vi "Dashboard Main.vi"() -> ()   [LabVIEW 2013]
uses:
  <vilib>/Rock Robotics/WPI/Camera/WPI_CameraSettings Read MJPG.ctl
  <vilib>/Rock Robotics/WPI/Camera/WPI_CameraImageSize.ctl
  <vilib>/event_ctls.llb/eventvkey.ctl
panel:
  in  "Mode":T1(ring)=enum."Auto Disabled"
  out "Encoder Speed":dbl(graph)
  in  "Rec Mode":enum32{"Stop", "Record", "Playback"}(radio)
  out "Battery":sgl
  out "High Gear":bool
  out "Speed":dbl(knob) scale=0.0..25.0
  out "Dashboard Connected":bool
  in  "Tab Control":T2(tab)
  in  "Autonmous To Run":string(combo)
  in  "Autonmous mode":string
  in  "Editable":bool
  in  "Reload Autonmous text file":bool
  in  "Save Auto file back to text file":bool
  out "Camera":T3(plugin-control)
  in  "Reload Constants":bool
  out "Variable Names":string[](array[string])
  out "Array of Numbers":dbl[](array[numeric])
  in  "Listbox":i32(listbox)
  in  "Reset Gyro":bool
  out "gyroAngle":dbl
  # "CHANGE IP!!!!!!!!!!!!!!!!!!!!!!"
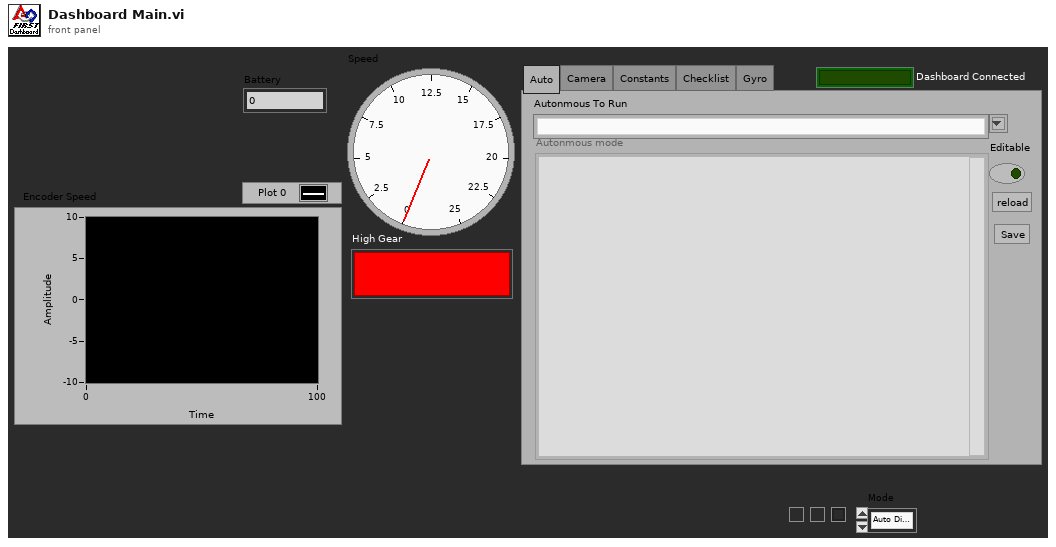
[diagram p1: front panel]
types:
  T1 = enum8{"Tele-Op Disabled", "Tele-Op Enabled", "Auto Disabled", "Auto Enabled", "Test Disabled", "Test Enabled", ""}
  T2 = enum32{"Auto", "Camera", "Constants", "Checklist", "Gyro"}
  T3 = typedef "IMAQ Image.ctl" = refnum<image>
  T4 = enum16{"None", "On Hover", "On Key Focus", "On Hover or Key Focus"}
  T5 = enum8{"Enabled", "Disabled", "Disabled and Grayed Out"}
  T6 = typedef "WPI_CameraSettings Read MJPG.ctl" = cluster{"fps":i32, "compression":i32, "Image Size":T7}
  T7 = typedef "WPI_CameraImageSize.ctl" = enum16{"640x480", "320x240", "160x120"}
  T8 = typedef "Image Type" = u32
  T9 = cluster{cluster{dbl, dbl}, cluster{dbl, dbl}, cluster{dbl, dbl}}
  T10 = cluster{"Digital Inputs":bool[], "Digital Outputs":bool[]}
  T11 = cluster{"Competition mode":bool, "Robot Link":bool, "Autonomous":bool, "Enabled":bool, "E-Stop":bool, "Simulated":bool, "TestMode":bool, "Docked Window":bool}
  T12 = typedef "eventvkey.ctl" = enum16{"ASCII", "Enter", "Return", "Shift", "Ctrl", "Alt", "Cmd", "Opt", "Caps", "NumLock", "Clear", "Break", "Up", "Down", "Left", "Right", "Insert", "Delete", "Home", "End", "PageUp", "PageDown", "Escape", "Help", "Pause", "ScrollLock", "F1", "F2", "F3", "F4", "F5", "F6", "F7", "F8", "F9", "F10", "F11", "F12", "F13", "F14", "F15", "F16", "F17", "F18", "F19", "F20", "F21", "F22", "F23", "F24", "Play", "VolumeUp", "VolumeDown", "Mute", "Two Byte Char"}
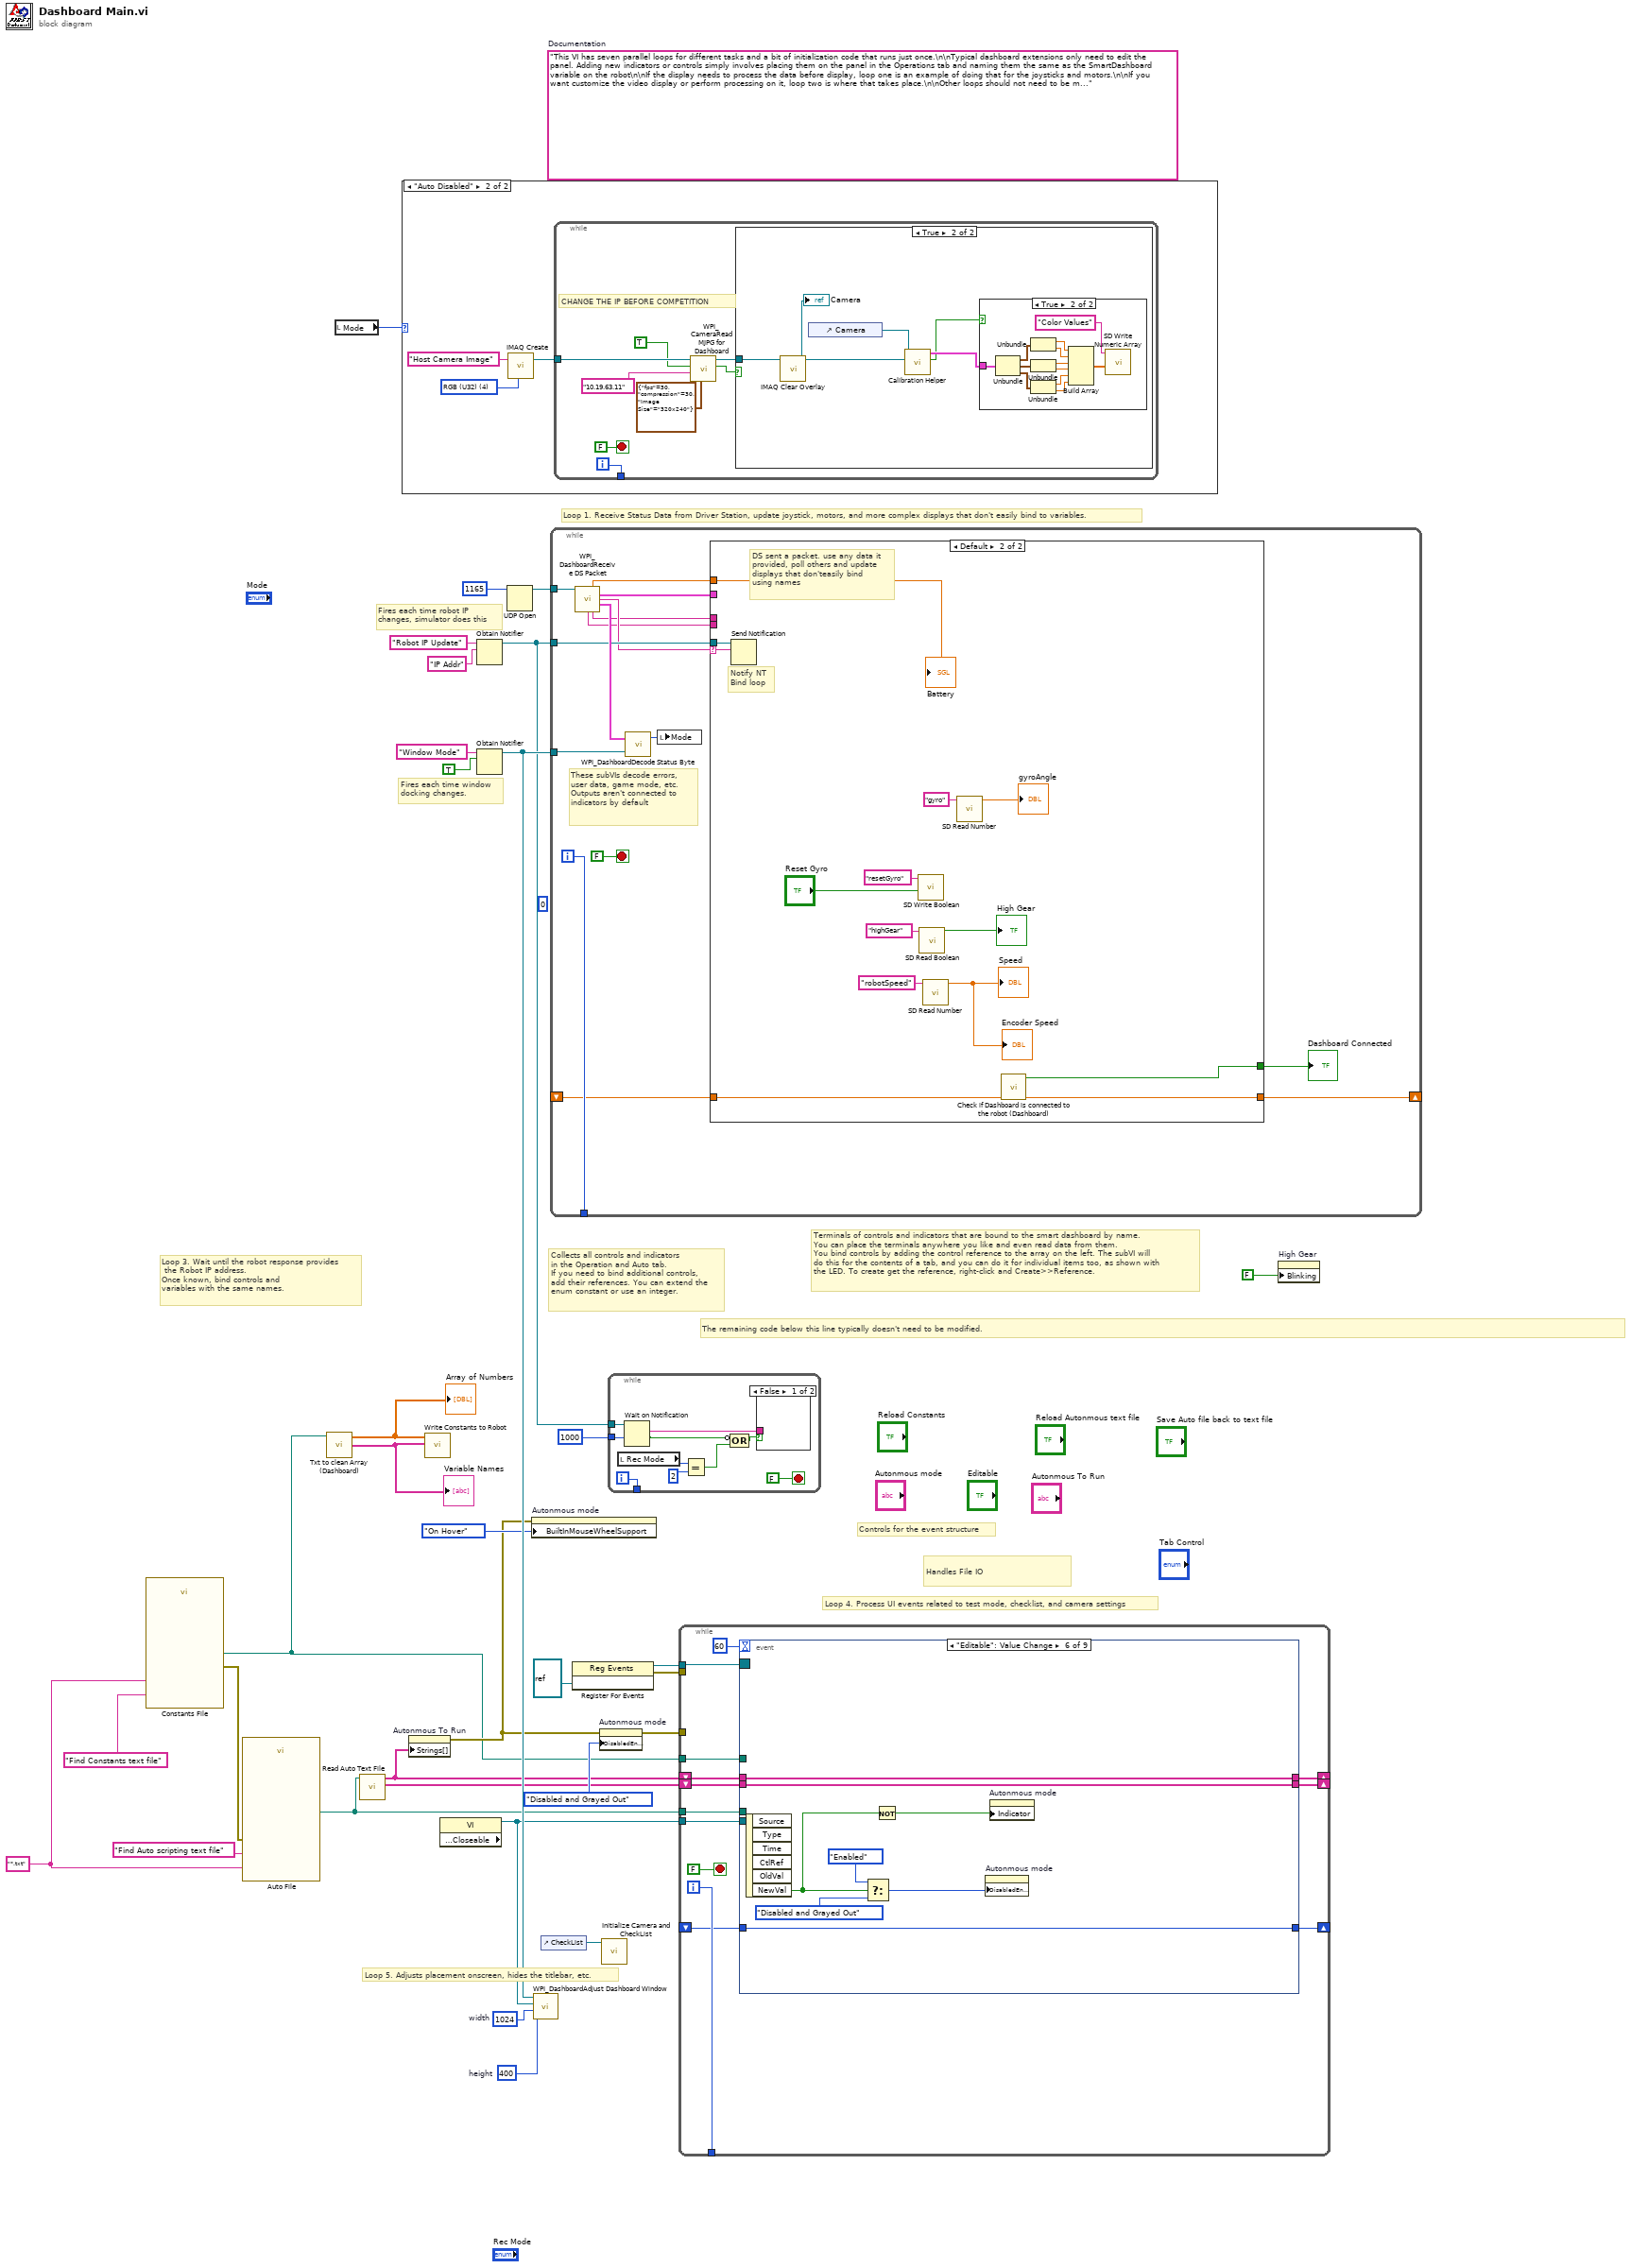
[diagram p0: block diagram]
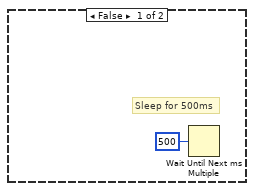
[diagram p3: hidden frame]
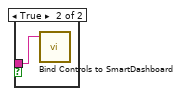
[diagram p5: hidden frame]
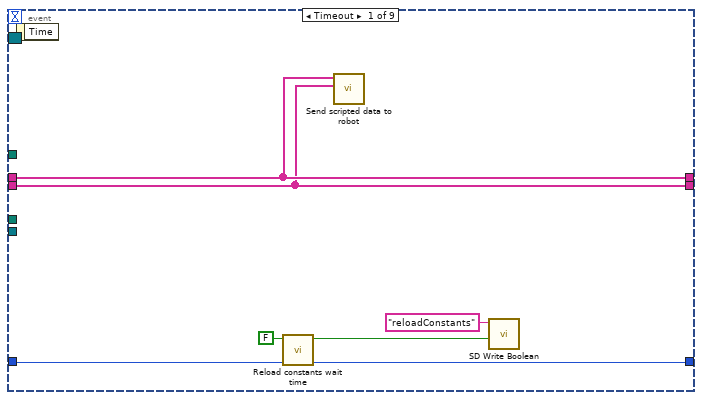
[diagram p6: hidden frame]
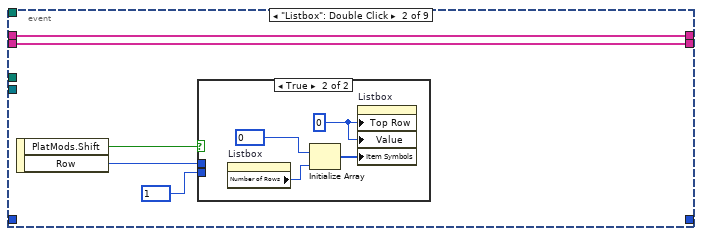
[diagram p7: hidden frame]
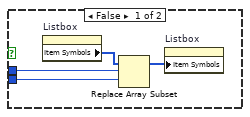
[diagram p8: hidden frame]
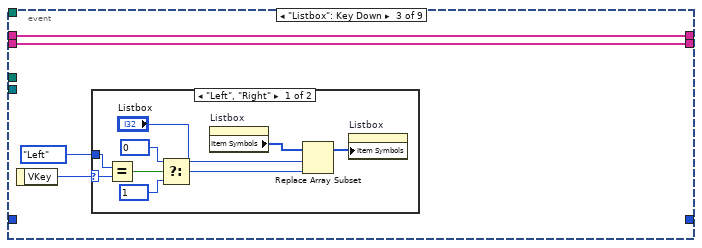
[diagram p9: hidden frame]
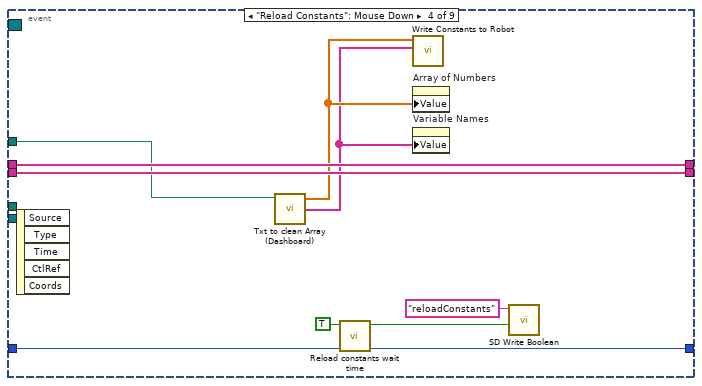
[diagram p11: hidden frame]
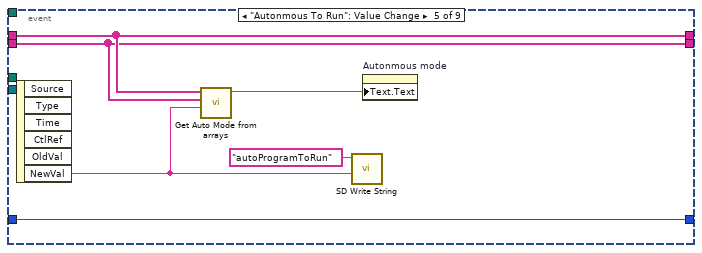
[diagram p12: hidden frame]
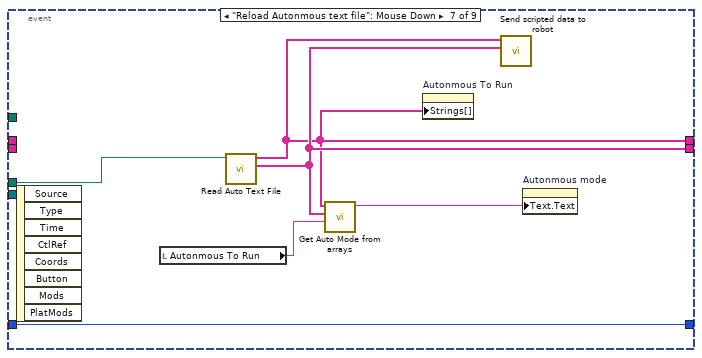
[diagram p13: hidden frame]
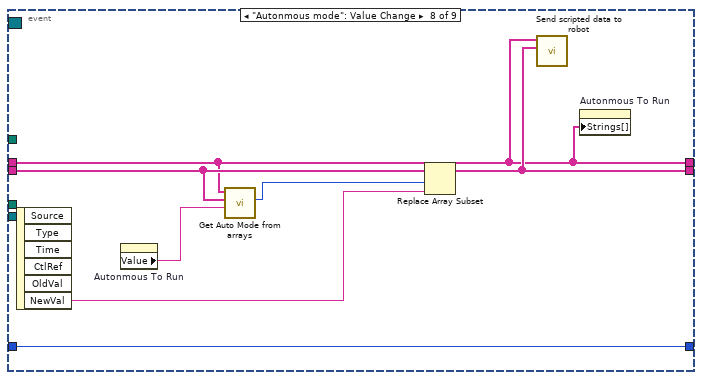
[diagram p14: hidden frame]
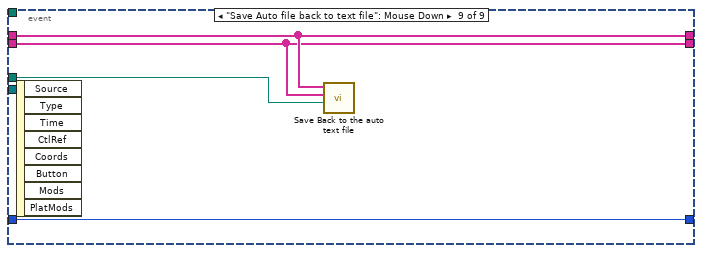
[diagram p15: hidden frame]
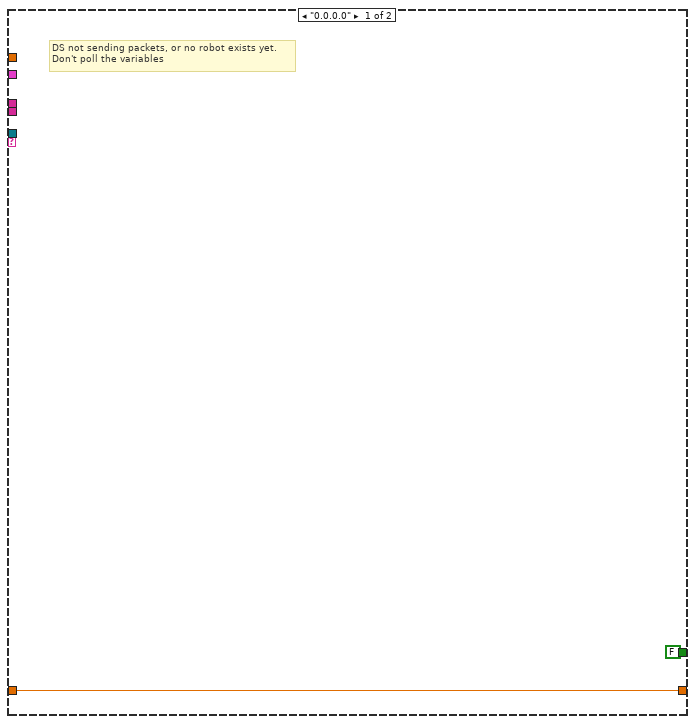
[diagram p16: hidden frame]
diagram:
  (unwired) u32 0 ("millisecond timer value out")
  w8 = "*.txt" ("pattern label")
  w22 = 400  # height
  w23 = 1024  # width
  (unwired) "This VI has seven parallel loops for different tasks and a bit of initialization code that runs just once.\n\nTypical dashboard extensions only need to edit the panel. Adding new indicators or controls simply involves placing them on the panel in the Operations tab and naming them the same as the SmartDashboard variable on the robot\n\nIf the display needs to process the data before display, loop one is an example of doing that for the joysticks and motors.\n\nIf you want customize the video display or perform processing on it, loop two is where that takes place.\n\nOther loops should not need to be modified. They are pretty standard, and document the task they perform."  # Documentation
  # "Loop 3. Wait until the robot response provides\n the Robot IP address.\nOnce known, bind controls and\nvariables with the same names."
  # "Controls for the event structure"
  # "Handles File IO"
  # "Fires each time robot IP\nchanges, simulator does this"
  # "Fires each time window\ndocking changes."
  # "Collects all controls and indicators\nin the Operation and Auto tab.\nIf you need to bind additional controls,\nadd their references. You can extend the\nenum constant or use an integer."
  # "The remaining code below this line typically doesn't need to be modified."
  # "Loop 4. Process UI events related to test mode, checklist, and camera settings"
  # "Terminals of controls and indicators that are bound to the smart dashboard by name.\nYou can place the terminals anywhere you like and even read data from them.\nYou bind controls by adding the control reference to the array on the left. The subVI will\ndo this for the contents of a tab, and you can do it for individual items too, as shown with\nthe LED. To create get the reference, right-click and Create>>Reference."
  # "Loop 5. Adjusts placement onscreen, hides the titlebar, etc."
  # "Loop 1. Receive Status Data from Driver Station, update joystick, motors, and more complex displays that don't easily bind to variables."
  n1 = call "Constants File"("prompt"="Find Constants text file", "pattern (all files)"=w8) -> ("selected path"=w11:path, "error out"=w10:errorcluster)  [unwired: 10 in, 2 out]
  n2 = call "Auto File"("prompt"="Find Auto scripting text file", "error in"=w10, "pattern (all files)"=w8) -> ("selected path"=w18:path)  [unwired: 9 in, 3 out]
  n3 = call "Txt to clean Array (Dashboard).vi"("file path"=w11) -> ("Variable Names"=w5:string[], "Array of Numbers"=w6:dbl[])  [unwired: 3 in, 1 out]
  "Array of Numbers" <- w6
  "Variable Names" <- w5
  n4 = local read "Mode"() -> (w1:T1)
  n5 = call "Read Auto Text File.vi"("selected path"=w18) -> ("Programs"=w15:string[], "Program Name"=w16:string[])  [unwired: 8 in, 1 out]
  n6 = case shown="\"Auto Disabled\"" w1 {
    frame "Tele-Op Disabled", Default {
    }
    frame "Auto Disabled" {
      w33 = T8 4 items=["Grayscale (U8)", "Grayscale (I16)", "Grayscale (SGL)", "Complex (CSG)", "RGB (U32)", "HSL (U32)", "RGB (U64)"] ("Image Type")
      n7 = call "IMAQ Create"("Image Name"="Host Camera Image", "Image Type"=w33) -> ("New Image"=w35:T3)  [unwired: 2 in, 2 out]
      n8 = while {
        tunnel: w35 -> [w41]
        tunnel: [w42] -> _
        i -> [w42]
        stop <- FALSE stop-if-true
        # "CHANGE THE IP BEFORE COMPETITION"
        n9 = call <vilib>:"WPI_CameraRead MJPG for Dashboard.vi"("Camera Settings"=T6 {"fps"=30, "compression"=30, "Image Size"=enum."320x240"}, "Camera IP"="10.19.63.11", "Enable"=TRUE, "Refnum in"=w41) -> ("Active"=w39:bool, "Refnum out"=w40:T3)  [unwired: 4 in, 2 out]
        n10 = case shown="True" w39 {
          tunnel: w40 -> [_ w45]
          frame False {
            # "Sleep for 500ms"
            n11 = Wait Until Next ms Multiple(millisecond multiple=u32 500) -> ()  [unwired: 1 out]
          }
          frame True {
            n12 = call "IMAQ Clear Overlay"("Image"=w45) -> ("Image Out"=w46:T3)  [unwired: 9 in, 1 out]
            "Camera" <- w46
            n13 = control-ref of="Camera"() -> (w47:refnum<vi>)
            n14 = call "Calibration Helper.vi"("Image"=w46, "Image Ctl Refnum"=w47) -> ("Changed"=w48:bool, "output color"=w49:T9)  [unwired: 8 in]
            n15 = case shown="True" w48 {
              tunnel: w49 -> [_ w50]
              frame False {
              }
              frame True {
                n16 = Unbundle(w50) -> (w59:cluster{dbl, dbl}, w61:cluster{dbl, dbl}, w60:cluster{dbl, dbl})
                n17 = Unbundle(w59) -> (w58:dbl, w57:dbl)
                n18 = Unbundle(w61) -> (w56:dbl, w55:dbl)
                n19 = Unbundle(w60) -> (w54:dbl, w53:dbl)
                n20 = Build Array(w58, w57, w56, w55, w54, w53) -> (w52:dbl[])
                n21 = call <vilib>:"SD Write Numeric Array.vi"("Numeric Array"=w52, "Name"="Color Values") -> ()  [unwired: 8 in, 2 out]
              }
            }
          }
        }
      }
    }
  }
  n22 = property on="Autonmous To Run" class="CmbBox"("Strings[]"=w16) -> (error out=w13:errorcluster)  [unwired: 2 in, 1 out]
  n23 = call "Write Constants to Robot.vi"("Variable Names"=w5, "Array of Numbers"=w6) -> ()  [unwired: 10 in]
  n24 = property class="VI" props=["Front Panel.Closeable"]() -> (reference out=w19:refnum<vi>)  [unwired: 2 in, 2 out]
  n25 = Obtain Notifier(name (unnamed)="Robot IP Update", notification data type="IP Addr" ("name (unnamed)")) -> (notifier out=w2:refnum<notifier>)  [unwired: 2 in, 2 out]
  n26 = Obtain Notifier(name (unnamed)="Window Mode", notification data type=TRUE) -> (notifier out=w21:refnum<notifier>)  [unwired: 2 in, 2 out]
  n27 = UDP Open(11:u16 1165 ("port")) -> (port=w31:refnum<k16>)  [unwired: 2 in, 4 out]
  n28 = property on="Autonmous mode" class="Str"(error in=w13, "BuiltInMouseWheelSupport"=T4."On Hover" ("Built-In Mouse Wheel Support")) -> ()  [unwired: 1 in, 2 out]
  n29 = call <vilib>:"WPI_DashboardAdjust Dashboard Window.vi"("height"=w22, "width"=w23, "reference in"=w19, "Notifier in"=w21) -> ()  [unwired: 8 in]
  n30 = control-ref of="CheckList"() -> (w20:refnum<vi>)
  n31 = while {
    tunnel: w31 -> [w74]
    tunnel: w2 -> [w71]
    tunnel: w21 -> [w73]
    tunnel: [w72] -> _
    shift-right: [w65] -> _
    shift-left: _ -> [w64]
    i -> [w72]
    stop <- FALSE stop-if-true
    # "These subVIs decode errors, user data, game mode, etc.\nOutputs aren't connected to indicators by default"
    n32 = call <vilib>:"WPI_DashboardReceive DS Packet.vi"("Recv Socket"=w74) -> ("Battery"=w66:sgl, "Driver Station"=w67:T10, "Robot IP Address"=w70:string, "Status"=w75:T11, "Low Priority User Data"=w69:string, "High Priority User Data"=w68:string)  [unwired: 1 in, 8 out]
    n33 = call <vilib>:"WPI_DashboardDecode Status Byte.vi"("Window Mode Notifier"=w73, "Status"=w75) -> ("Mode"=w62:T1)  [unwired: 1 out]
    n34 = local write "Mode"(w62) -> ()
    n35 = case shown="Default" w70 {
      selector: w70 -> [_ w91]
      tunnel: w71 -> [_ w92]
      tunnel: w69 -> [_ _]
      tunnel: w68 -> [_ _]
      tunnel: w67 -> [_ _]
      tunnel: w66 -> [_ w85]
      tunnel: [w78 w90] -> w65
      tunnel: w64 -> [w78 w89]
      tunnel: [FALSE ("Number Changing") w84] -> w63
      frame "0.0.0.0" {
        # "DS not sending packets, or no robot exists yet.\nDon't poll the variables"
      }
      frame Default {
        # "Notify NT\nBind loop"
        # "DS sent a packet. use any data it\nprovided, poll others and update\ndisplays that don'teasily bind\nusing names"
        n36 = Send Notification(notification=w91, notifier=w92) -> ()  [unwired: 1 in, 2 out]
        n37 = call <vilib>:"SD Write Boolean.vi"("Boolean"="Reset Gyro", "Name"="resetGyro") -> ()  [unwired: 8 in, 2 out]
        n38 = call <vilib>:"SD Read Boolean.vi"("Name"="highGear") -> ("Boolean"=→"High Gear":bool)  [unwired: 8 in, 2 out]
        n39 = call <vilib>:"SD Read Number.vi"("Name"="robotSpeed") -> ("Numeric"=→"Speed" →"Encoder Speed":dbl)  [unwired: 8 in, 2 out]
        n40 = call <vilib>:"SD Read Number.vi"("Name"="gyro") -> ("Numeric"=→"gyroAngle":dbl)  [unwired: 8 in, 2 out]
        n41 = call "Check if Dashboard is connected to the robot (Dashboard).vi"("From shift"=w89) -> ("to shift"=w90:dbl, "Number Changing"=w84:bool)  [unwired: 9 in]
        "Battery" <- w85
      }
    }
    "Dashboard Connected" <- w63
  }
  n42 = register-events(refnum<vi> refnum) -> (reference out=w26:refnum<event-registration>, error out=w25:errorcluster)  [unwired: 2 in]
  n43 = property on="Autonmous mode" class="Str"(error in=w13, "DisabledEnum"=T5."Disabled and Grayed Out" ("Disabled")) -> (error out=w12:errorcluster)  [unwired: 1 in, 1 out]
  n44 = call "Initialize Camera and CheckList.vi"("ListBox in"=w20) -> ()  [unwired: 11 in]
  n45 = while {
    tunnel: w2 -> [w101]
    tunnel: [w99] -> _
    tunnel: u32 1000 ("milliseconds to wait") -> [w98]
    i -> [w99]
    stop <- FALSE stop-if-true
    n46 = local read "Rec Mode"() -> (w94:enum32{"Stop", "Record", "Playback"})
    n47 = Wait on Notification(notifier=w101, timeout in ms (-1)=w98) -> (notification=w100:string, timed out?=w96:bool)  [unwired: 2 in, 2 out]
    n48 = Equal?(x=w94, y=u16 2 ("Rec Mode")) -> (x = y?=w95:bool)
    n49 = Compound Arithmetic op=OR(invert w96, w95) -> (w97:bool)
    n50 = case shown="False" w97 {
      tunnel: w100 -> [_ w103]
      frame False {
      }
      frame True {
        n51 = call <vilib>:"Bind Controls to SmartDashboard.vi"("Server IP Address"=w103) -> ()  [unwired: 11 in]
      }
    }
  }
  n52 = while {
    tunnel: [w114] -> _
    tunnel: w26 -> [w113]
    tunnel: w25 -> [_]
    tunnel: w19 -> [w112]
    tunnel: w18 -> [w111]
    tunnel: w11 -> [w110]
    shift-right: [w107] -> _
    shift-left: w16 -> [w109]
    shift-right: [w106] -> _
    shift-left: w15 -> [w108]
    tunnel: w12 -> [_]
    shift-right: [w105] -> _
    shift-left: _ -> [w104]
    i -> [w114]
    stop <- FALSE stop-if-true
    n53 = event shown="[5] \"Editable\": Value Change" {
      selector: w113 -> [_ _ _ _ _ _ _ _ _]
      dyn-events: _ -> [_ _ _ _ _ _ _ _ _]
      timeout: u32 60 ("milliseconds to wait") -> [_ _ _ _ _ _ _ _ _]
      tunnel: w112 -> [_ _ _ _ _ _ _ _ _]
      tunnel: w111 -> [_ _ _ _ _ _ w179 _ w188]
      tunnel: w110 -> [_ _ _ w157 _ _ _ _ _]
      tunnel: w108 -> [w122 w124 w137 w158 w161 w167 _ w185 w189]
      tunnel: w109 -> [w123 w125 w138 w159 w162 w168 _ w182 w190]
      tunnel: [w123 w125 w138 w159 w162 w168 w175 w182 w190] -> w107
      tunnel: [w122 w124 w137 w158 w161 w167 w178 w183 w189] -> w106
      tunnel: [w120 _ _ w153 w160 w166 w174 w180 w187] -> w105
      tunnel: w104 -> [w121 _ _ w154 w160 w166 w174 w180 w187]
      event Timeout {
        n54 = event-data() -> ()  [unwired: 1 in, 1 out]
        n55 = call "Reload constants wait time.vi"("millisecond timer value in"=w121, "Reload Constants"=FALSE) -> ("millisecond timer value out"=w120:u32, "Tell Robot to reload constants"=w117:bool)  [unwired: 8 in]
        n56 = call "Send scripted data to robot.vi"("Programs"=w122, "Program Name"=w123) -> ()  [unwired: 10 in]
        n57 = call <vilib>:"SD Write Boolean.vi"("Boolean"=w117, "Name"="reloadConstants") -> ()  [unwired: 8 in, 2 out]
      }
      event "Listbox": Double Click {
        n58 = event-data() -> ("PlatMods.Shift"=w126:bool, "Row"=w128:i32)  [unwired: 1 in]
        n59 = case shown="True" w126 {
          tunnel: w128 -> [w132 _]
          tunnel: 1 -> [w131 _]
          frame False {
            n60 = property on="Listbox" class="LstBox (strict)"() -> ("Item Symbols"=w130:i32[])  [unwired: 2 in, 2 out]
            n61 = Replace Array Subset(array=w130, new element=w131, index=w132) -> (w129:i32[])
            n62 = property on="Listbox" class="LstBox (strict)"("Item Symbols"=w129) -> ()  [unwired: 2 in, 2 out]
          }
          frame True {
            w133 = 0 ("Top Row")
            n63 = property on="Listbox" class="LstBox (strict)"() -> ("Number of Rows"=w135:u32)  [unwired: 2 in, 2 out]
            n64 = Initialize Array(0, w135) -> (w134:i32[])
            n65 = property on="Listbox" class="LstBox (strict)"("Top Row"=w133, "Value"=w133, "Item Symbols"=w134) -> ()  [unwired: 2 in, 2 out]
          }
        }
      }
      event "Listbox": Key Down {
        n66 = event-data() -> ("VKey"=w140:T12)  [unwired: 1 in]
        n67 = case shown="\"Left\", \"Right\"" w140 {
          selector: w140 -> [w145 _]
          tunnel: eventvkey."Left" ("VKey") -> [w143 _]
          frame "Left", "Right" {
            n68 = Equal?(x=w143, y=w145) -> (x = y?=w144:bool)
            n69 = Select(t=0, s=w144, f=1) -> (s? t:f=w146:i32)
            n70 = property on="Listbox" class="LstBox (strict)"() -> ("Item Symbols"=w149:i32[])  [unwired: 2 in, 2 out]
            n71 = Replace Array Subset(array=w149, new element=w146, index="Listbox") -> (w148:i32[])
            n72 = property on="Listbox" class="LstBox (strict)"("Item Symbols"=w148) -> ()  [unwired: 2 in, 2 out]
          }
          frame Default {
          }
        }
      }
      event "Reload Constants": Mouse Down {
        n73 = event-data() -> ()  [unwired: 1 in, 5 out]
        n74 = call "Txt to clean Array (Dashboard).vi"("file path"=w157) -> ("Variable Names"=w155:string[], "Array of Numbers"=w156:dbl[])  [unwired: 3 in, 1 out]
        n75 = call "Reload constants wait time.vi"("millisecond timer value in"=w154, "Reload Constants"=TRUE) -> ("millisecond timer value out"=w153:u32, "Tell Robot to reload constants"=w150:bool)  [unwired: 8 in]
        n76 = call "Write Constants to Robot.vi"("Variable Names"=w155, "Array of Numbers"=w156) -> ()  [unwired: 10 in]
        n77 = property on="Array of Numbers" class="Arr (strict)"("Value"=w156) -> ()  [unwired: 2 in, 2 out]
        n78 = property on="Variable Names" class="Arr (strict)"("Value"=w155) -> ()  [unwired: 2 in, 2 out]
        n79 = call <vilib>:"SD Write Boolean.vi"("Boolean"=w150, "Name"="reloadConstants") -> ()  [unwired: 8 in, 2 out]
      }
      event "Autonmous To Run": Value Change {
        n80 = event-data() -> ("NewVal"=w164:string)  [unwired: 1 in, 5 out]
        n81 = call "Get Auto Mode from arrays.vi"("Auto Name"=w164, "Programs"=w161, "Program Name"=w162) -> ("Auto Program"=w163:string)  [unwired: 7 in, 1 out]
        n82 = call <vilib>:"SD Write String.vi"("String"=w164, "Name"="autoProgramToRun") -> ()  [unwired: 8 in, 2 out]
        n83 = property on="Autonmous mode" class="Str"("Text.Text"=w163) -> ()  [unwired: 2 in, 2 out]
      }
      event "Editable": Value Change {
        n84 = event-data() -> ("NewVal"=w170:bool)  [unwired: 1 in, 5 out]
        n85 = Select(t=T5."Enabled" ("Disabled"), s=w170, f=T5."Disabled and Grayed Out" ("Disabled")) -> (s? t:f=w171:T5)
        n86 = Not(x=w170) -> (.not. x?=w169:bool)
        n87 = property on="Autonmous mode" class="Str"("DisabledEnum"=w171) -> ()  [unwired: 2 in, 2 out]
        n88 = property on="Autonmous mode" class="Str"("Indicator"=w169) -> ()  [unwired: 2 in, 2 out]
      }
      event "Reload Autonmous text file": Mouse Down {
        n89 = event-data() -> ()  [unwired: 1 in, 8 out]
        n90 = local read "Autonmous To Run"() -> (w177:string)
        n91 = call "Read Auto Text File.vi"("selected path"=w179) -> ("Programs"=w178:string[], "Program Name"=w175:string[])  [unwired: 8 in, 1 out]
        n92 = call "Get Auto Mode from arrays.vi"("Auto Name"=w177, "Programs"=w178, "Program Name"=w175) -> ("Auto Program"=w176:string)  [unwired: 7 in, 1 out]
        n93 = property on="Autonmous To Run" class="CmbBox"("Strings[]"=w175) -> ()  [unwired: 2 in, 2 out]
        n94 = call "Send scripted data to robot.vi"("Programs"=w178, "Program Name"=w175) -> ()  [unwired: 10 in]
        n95 = property on="Autonmous mode" class="Str"("Text.Text"=w176) -> ()  [unwired: 2 in, 2 out]
      }
      event "Autonmous mode": Value Change {
        n96 = event-data() -> ("NewVal"=w181:string)  [unwired: 1 in, 5 out]
        n97 = property on="Autonmous To Run" class="CmbBox"() -> ("Value"=w186:string)  [unwired: 2 in, 2 out]
        n98 = call "Get Auto Mode from arrays.vi"("Auto Name"=w186, "Programs"=w185, "Program Name"=w182) -> ("index"=w184:i32)  [unwired: 7 in, 1 out]
        n99 = Replace Array Subset(array=w185, new element=w181, index=w184) -> (w183:string[])
        n100 = call "Send scripted data to robot.vi"("Programs"=w183, "Program Name"=w182) -> ()  [unwired: 10 in]
        n101 = property on="Autonmous To Run" class="CmbBox"("Strings[]"=w182) -> ()  [unwired: 2 in, 2 out]
      }
      event "Save Auto file back to text file": Mouse Down {
        n102 = event-data() -> ()  [unwired: 1 in, 8 out]
        n103 = call "Save Back to the auto text file.vi"("Path"=w188, "Programs"=w189, "Program Name"=w190) -> ()  [unwired: 9 in]
      }
    }
  }
  n104 = property on="High Gear" class="Bool (strict)"("Blinking"=FALSE) -> ()  [unwired: 2 in, 2 out]
